vi "DAQmx Create Channel (AI-Frequency-Voltage).vi"(0 "task in":refnum<k21>, 1 "maximum value":dbl=100.0 format="%0.2f", 2 "minimum value":dbl=1.0 format="%0.2f", 5 "physical channels":tag, 6 "threshold level":dbl format="%0.2f", 7 "name to assign":string, 8 "hysteresis":dbl format="%.2f", 9 "units":i32(ring)=10373 items=["Hz"=10373, "From Custom Scale"=10065], 11 "error in":errorcluster, 12 "custom scale name":tag) -> (4 "task out":refnum<k21>, 15 "error out":errorcluster)   [LabVIEW 2011]
doc: "Creates channel(s) that use a frequency-to-voltage converter to measure frequency."
uses:
  C:/Program Files/National Instruments/LabVIEW 2011/resource/objmgr/daqmx.rc
panel:
  # "input limits"
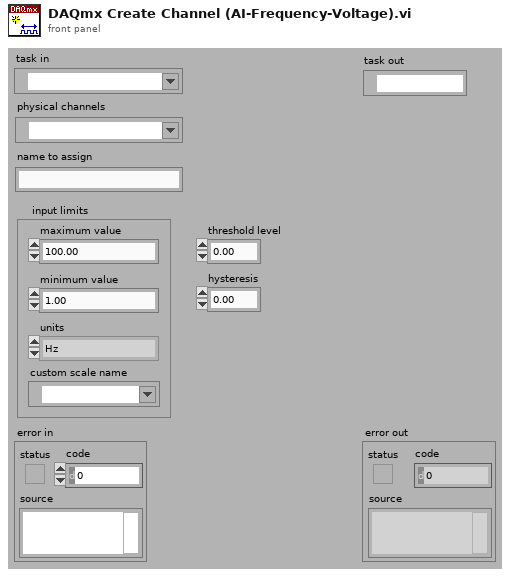
[diagram p1: front panel]
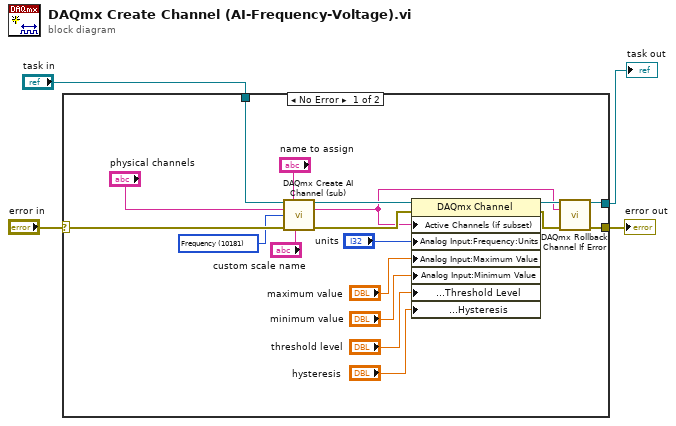
[diagram p0: block diagram]
diagram:
  n1 = case shown="No Error" "error in" {
    selector: "error in" -> [w21 w24]
    tunnel: [w6 w24] -> w4
    tunnel: "task in" -> [w22 w23]
    tunnel: [w7 w23] -> w1
    frame No Error {
      w14 = 10181 items=["Voltage"=10322, "Current"=10134, "More:Voltage:Custom with Excitation"=10323, "More:Current:Custom with Excitation"=10136, "Frequency"=10181, "Period"=10257, "Resistance"=10278, "Temperature:Thermocouple"=10303, "Temperature:Thermistor"=10302, "Temperature:RTD"=10301, "Temperature:Built-in Sensor"=10311, "Strain Gage"=10300] ("measurement type")
      n2 = call "DAQmx Create AI Channel (sub).vi"("task in"=w22, "virtual channel name"="name to assign", "physical channel name"="physical channels", "measurement type"=w14, "error in"=w21, "custom scale"="custom scale name") -> ("task out"=w10:refnum<k21>, "channel names"=w5:string, "error out"=w18:errorcluster)  [unwired: 7 out]
      n3 = property class="DAQmx Channel"(reference=w10, error in=w18, "Active Channels (if subset)"=w5, "Analog Input:Frequency:Units"="units", "Analog Input:Maximum Value"="maximum value", "Analog Input:Minimum Value"="minimum value", "Analog Input:Frequency:Voltage:Threshold Level"="threshold level", "Analog Input:Frequency:Voltage:Hysteresis"="hysteresis") -> (reference out=w9:refnum<k21>, error out=w8:errorcluster)
      n4 = call "DAQmx Rollback Channel If Error.vi"("task in"=w9, "channel names"=w5, "error in"=w8) -> ("task out"=w7:refnum<k21>, "error out"=w6:errorcluster)  [unwired: 11 out]
    }
    frame Error {
    }
  }
  "error out" <- w4
  "task out" <- w1
